vi "test Parse DBL Array1.vi"(11 "Test Case In":refnum<class "Test Named Fields Parser.lvclass">) -> (0 "error out":errorcluster, 3 "Test Case Out":refnum<class "Test Named Fields Parser.lvclass">)   [LabVIEW 2024, in "Test Named Fields Parser.lvclass"]
uses:
  Test Named Fields Parser.lvclass
  C:/Program Files/National Instruments/LabVIEW 2025/vi.lib/Astemes/LUnit/Test Case.lvclass
  CSV Parser/Named Fields Parser/Named Fields Parser.lvclass
  <vilib>/Astemes/LUnit/Test Case.lvclass/Test Case.ctl
  4993e8ee-a06a-463a-9684-69129f64d5ce.vi
  <vilib>/Astemes/LUnit/Append Pass Result.vi
  <vilib>/Astemes/LUnit/Append Fail Result.vi
  4993e8ee-a06a-463a-9684-69129f64d5ce.vi/9c5d11cd-9439-4240-a1ee-d9baace9c924.vi
  <vilib>/Astemes/LUnit/Run In UI.vi
  <vilib>/Utility/error.llb/Clear Errors.vi
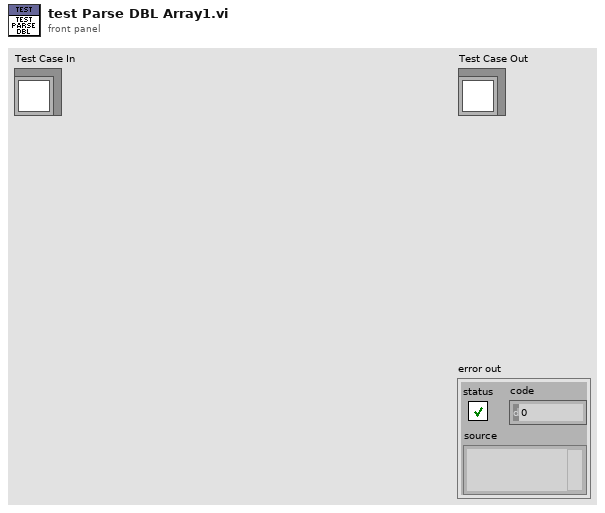
[diagram p1: front panel]
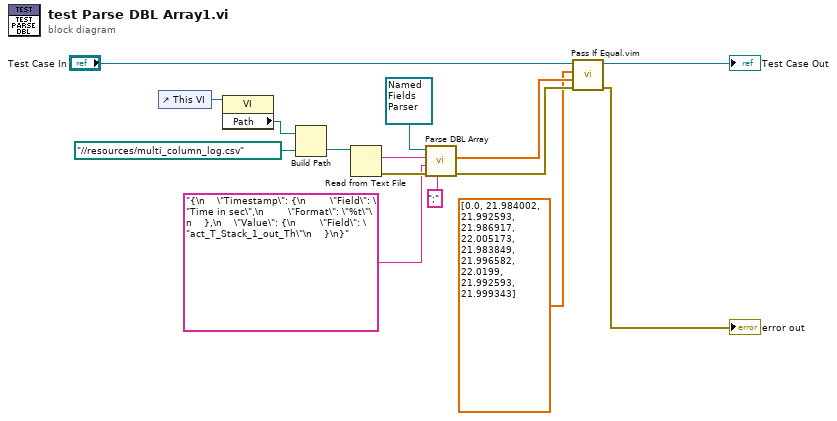
[diagram p0: block diagram]
diagram:
  n1 = control-ref of="This VI"() -> (w10:refnum<vi>)
  n2 = property class="VI"(reference=w10) -> ("Path"=w9:path)  [unwired: 1 in, 2 out]
  n3 = Build Path(base path=w9, name or relative path=path "../../resources/multi_column_log.csv" ("file (use dialog)")) -> (appended path=w12:path)
  n4 = Read from Text File(file (use dialog)=w12) -> (text=w8:string, error out=w7:errorcluster)  [unwired: 3 in, 2 out]
  n5 = call-dynamic "Parse DBL Array.vi"("Seperator"=";", "error in"=w7, "Input <JSON>"="{\n    \"Timestamp\": {\n        \"Field\": \"Time in sec\",\n        \"Format\": \"%t\"\n    },\n    \"Value\": {\n        \"Field\": \"act_T_Stack_1_out_Th\"\n    }\n}", "csv string"=w8, "Named Columns Parser in"=refnum<class "Named Fields Parser.lvclass"> refnum) -> ("error out"=w5:errorcluster, "DBL Array"=w2:dbl[])  [unwired: 4 in, 1 out]
  n6 = call "Pass If Equal.vim"("error in (no error)"=w5, "Actual"=w2, "Expected"=dbl[] [0.0, 21.984002, 21.992593, 21.986917, 22.005173, 21.983849, 21.996582, 22.0199, 21.992593, 21.999343] ("DBL Array"), "LUnit Test Case In"="Test Case In") -> ("error out"=→"error out":errorcluster, "LUnit Test Case Out"=→"Test Case Out":refnum<class "Test Named Fields Parser.lvclass">)  [unwired: 6 in]
